vi "Setup subWorker - Registration.vi"(8 "error in":errorcluster, 11 "gui in":refnum<class "gui.lvclass">) -> (0 "error out":errorcluster, 3 "gui out":refnum<class "gui.lvclass">)   [LabVIEW 2023, in "GUI.lvlib" / "gui.lvclass"]
doc: "This VI sets up the framework parameters of a statically-linked subWorker."
uses:
  gui.lvclass
  gui.lvclass/gui.ctl
  Registration Worker/Registration.lvclass
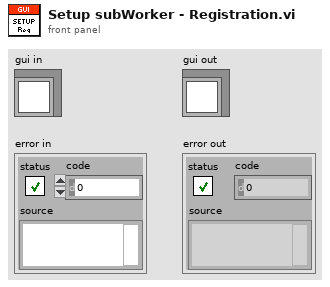
[diagram p1: front panel]
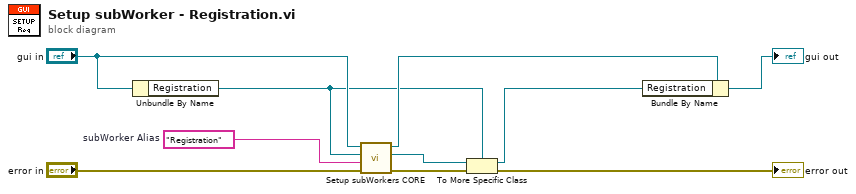
[diagram p0: block diagram]
diagram:
  w6 = "Registration"  # subWorker Alias
  n1 = Unbundle By Name("gui in") -> ("Registration"=w3:refnum<class "Registration.lvclass">)
  n2 = call-dynamic "Setup subWorkers CORE.vi"("error in"="error in", "subWorker Alias"=w6, "subWorker"=w3, "Worker"="gui in") -> ("error out"=w5:errorcluster, "subWorker out"=w1:refnum<class "Worker.lvclass">, "Worker out"=w8:refnum<class "gui.lvclass">)  [unwired: 5 in]
  n3 = To More Specific Class(target class=w3, reference=w1, error in=w5) -> (specific class reference=w2:refnum<class "Registration.lvclass">, error out=→"error out":errorcluster)
  n4 = Bundle By Name(cluster=w8, "Registration"=w2) -> (→"gui out":refnum<class "gui.lvclass">)
